vi "SysDef.Node.Info.Get.vi"(8 "error in (no error)":errorcluster, 10 "BaseNode Ref":refnum<k24>, 11 "NodeIDUtil Ref in":refnum<k24>) -> (0 "error out":errorcluster, 1 "Item Info":T1, 2 "BaseNode Ref out":refnum<k24>, 3 "NodeIDUtil Ref out":refnum<k24>)   [LabVIEW 2015, in "Advanced System Definition.lvlib"]
uses:
  SysDef API/Advanced System Definition.lvlib
  NationalInstruments.VeriStand.SystemStorage
  NationalInstruments.VeriStand.SystemDefinitionAPI
  _Types/TreeItem.Info.ctl
  <vilib>/NI Veristand/Custom Device API/Custom Device Channel.ctl
  <vilib>/NI Veristand/Custom Device API/Custom Device Channel Type.ctl
  <vilib>/NI Veristand/Custom Device API/Custom Device Waveform.ctl
  <vilib>/NI Veristand/Custom Device API/Custom Device Waveform DataType.ctl
  <vilib>/NI Veristand/Custom Device API/Custom Device API.lvlib
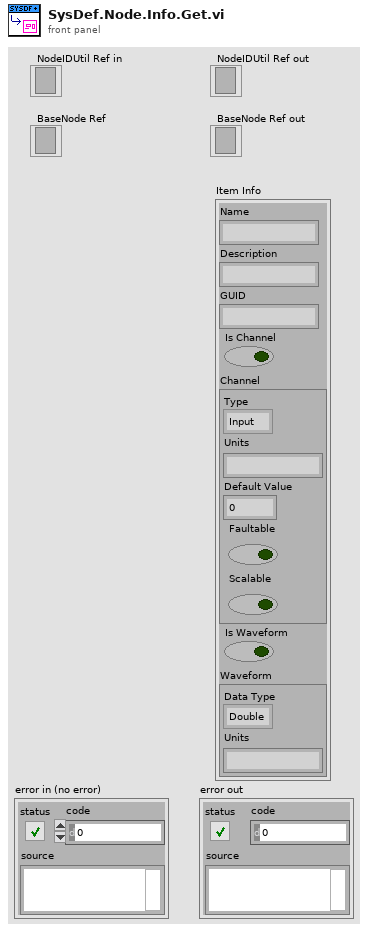
[diagram p1: front panel]
types:
  T1 = typedef "Advanced System Definition.lvlib/TreeItem.Info.ctl" = cluster{"Name":string, "Description":string, "GUID":string, "Is Channel":bool, "Channel":T2, "Is Waveform":bool, "Waveform":T4}
  T2 = typedef "Custom Device API.lvlib/Custom Device Channel.ctl" = cluster{"Type":T3, "Units":string, "Default Value":dbl, "Faultable":bool, "Scalable":bool}
  T3 = typedef "Custom Device API.lvlib/Custom Device Channel Type.ctl" = enum16{"Input", "Output"}
  T4 = typedef "Custom Device API.lvlib/Custom Device Waveform.ctl" = cluster{"Data Type":T5, "Units":string}
  T5 = typedef "Custom Device API.lvlib/Custom Device Waveform DataType.ctl" = enum16{"Double", "Complex Double"}
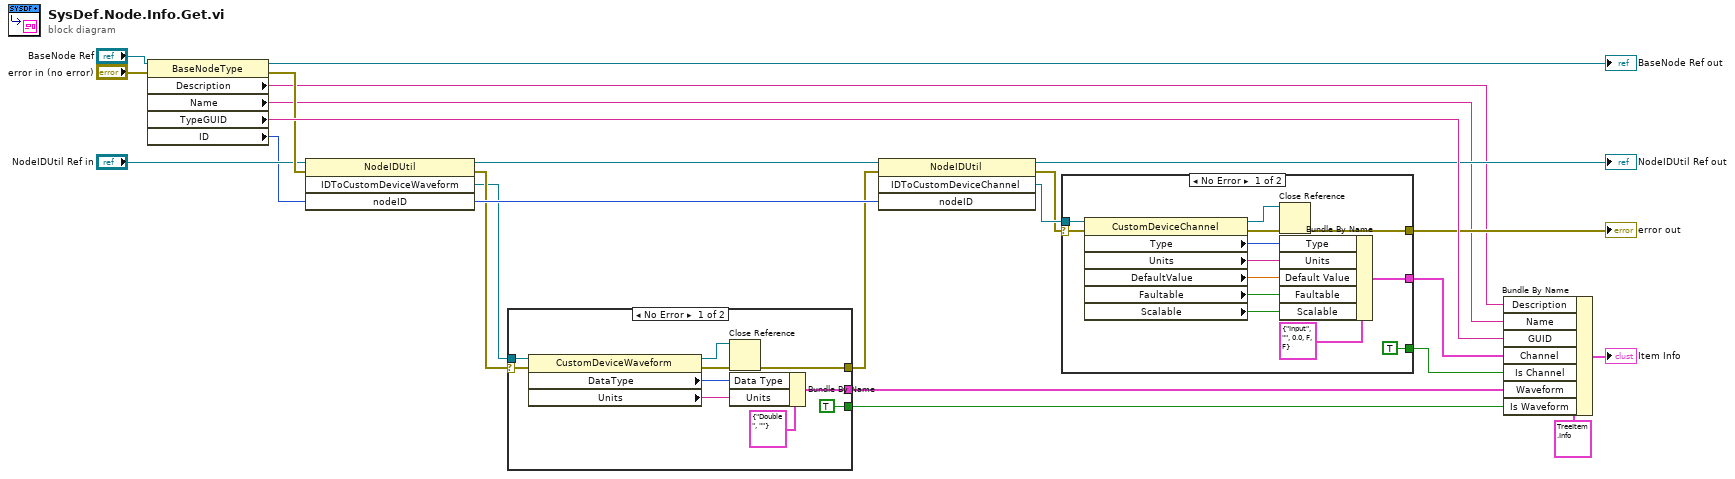
[diagram p0: block diagram]
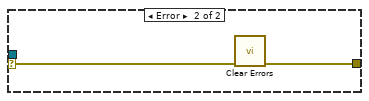
[diagram p2: hidden frame]
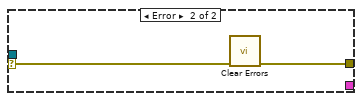
[diagram p3: hidden frame]
diagram:
  n1 = property class="BaseNodeType"(reference="BaseNode Ref", error in="error in (no error)") -> (reference out=→"BaseNode Ref out":refnum<k24>, error out=w19:errorcluster, "Description"=w9:string, "Name"=w6:string, "TypeGUID"=w21:string, "ID"=w17:u64)
  n2 = invoke class="NodeIDUtil" method="IDToCustomDeviceWaveform"(reference="NodeIDUtil Ref in", error in=w19, "nodeID"=w17) -> (reference out=w13:refnum<k24>, error out=w15:errorcluster, "IDToCustomDeviceWaveform"=w14:refnum<k24>)  [unwired: 1 in, 1 out]
  n3 = case shown="No Error" w15 {
    selector: w15 -> [w30 w35]
    tunnel: [w25 w34] -> w10
    tunnel: w14 -> [w29 _]
    tunnel: [TRUE _] -> w4
    tunnel: [w27 _] -> w8
    frame No Error {
      n4 = property class="CustomDeviceWaveform"(reference=w29, error in=w30) -> (reference out=w24:refnum<k24>, error out=w26:errorcluster, "DataType"=w32:i32, "Units"=w33:string)
      n5 = Close Reference(reference=w24, error in (no error)=w26) -> (error out=w25:errorcluster)
      n6 = Bundle By Name(cluster=T4 {"Data Type"=enum."Double", "Units"=""} ("Waveform"), "Data Type"=w32, "Units"=w33) -> (w27:T4)
    }
    frame Error {
      n7 = call <vilib>:"Clear Errors.vi"("error in (no error)"=w35) -> ("error out"=w34:errorcluster)  [unwired: 5 in, 1 out]
    }
  }
  n8 = invoke class="NodeIDUtil" method="IDToCustomDeviceChannel"(reference=w13, error in=w10, "nodeID"=w17) -> (reference out=→"NodeIDUtil Ref out":refnum<k24>, error out=w11:errorcluster, "IDToCustomDeviceChannel"=w12:refnum<k24>)  [unwired: 1 in, 1 out]
  n9 = case shown="No Error" w11 {
    selector: w11 -> [w41 w50]
    tunnel: [w36 w49] -> w16
    tunnel: [TRUE _] -> w5
    tunnel: w12 -> [w40 _]
    tunnel: [w39 _] -> w7
    frame No Error {
      n10 = property class="CustomDeviceChannel"(reference=w40, error in=w41) -> (reference out=w38:refnum<k24>, error out=w37:errorcluster, "Type"=w42:i32, "Units"=w44:string, "DefaultValue"=w45:dbl, "Faultable"=w46:bool, "Scalable"=w47:bool)
      n11 = Close Reference(reference=w38, error in (no error)=w37) -> (error out=w36:errorcluster)
      n12 = Bundle By Name(cluster=T2 {"Type"=enum."Input", "Units"="", "Default Value"=0.0, "Faultable"=FALSE, "Scalable"=FALSE} ("Channel"), "Type"=w42, "Units"=w44, "Default Value"=w45, "Faultable"=w46, "Scalable"=w47) -> (w39:T2)
    }
    frame Error {
      n13 = call <vilib>:"Clear Errors.vi"("error in (no error)"=w50) -> ("error out"=w49:errorcluster)  [unwired: 5 in, 1 out]
    }
  }
  "error out" <- w16
  n14 = Bundle By Name(cluster=T1 {"Name"="", "Description"="", "GUID"="", "Is Channel"=FALSE, "Channel"={"Type"=enum."Input", "Units"="", "Default Value"=0.0, "Faultable"=FALSE, "Scalable"=FALSE}, "Is Waveform"=FALSE, "Waveform"={"Data Type"=enum."Double", "Units"=""}} ("Item Info"), "Description"=w9, "Name"=w6, "GUID"=w21, "Channel"=w7, "Is Channel"=w5, "Waveform"=w8, "Is Waveform"=w4) -> (→"Item Info":T1)
